vi "Read Timeout (ms).vi"(8 "error in":errorcluster, 11 "EIP Tags Configuration in":refnum<class "EIP Tags Configuration.lvclass">) -> (0 "error out":errorcluster, 2 "Timeout (ms)":i32=1000, 3 "EIP Tags Configuration out":refnum<class "EIP Tags Configuration.lvclass">)   [LabVIEW 2013, in "EIP Tags Configuration.lvclass"]
uses:
  EIP Tags Configuration.lvclass
  EIP Tags Configuration.lvclass/EIP Tags Configuration.ctl
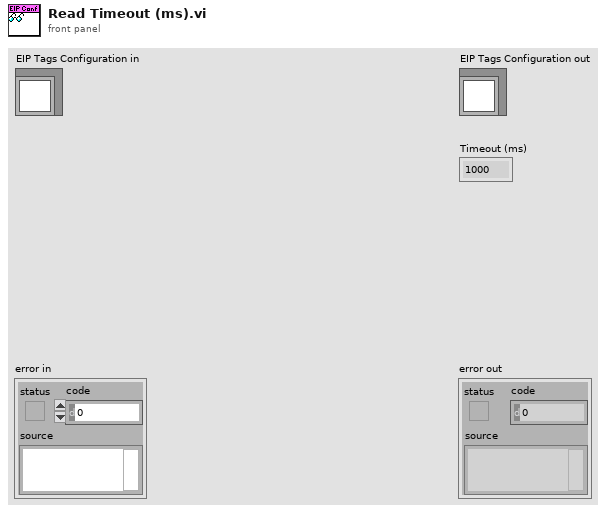
[diagram p1: front panel]
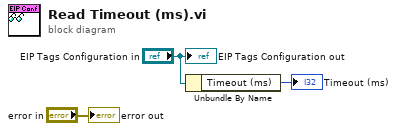
[diagram p0: block diagram]
diagram:
  n1 = Unbundle By Name("EIP Tags Configuration in") -> ("Timeout (ms)"=→"Timeout (ms)":i32)
  "error out" <- "error in"
  "EIP Tags Configuration out" <- "EIP Tags Configuration in"
